vi "for_v0_v0.vi"() -> ()   [LabVIEW 2009]
panel:
  out "Numeric":dbl
  # "Afisare numere 0-24"
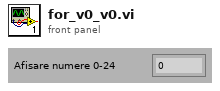
[diagram p1: front panel]
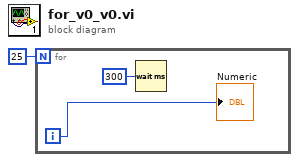
[diagram p0: block diagram]
diagram:
  n1 = for {
    N: 25 -> [_]
    i -> [w3]
    n2 = Wait (ms)(milliseconds to wait=u32 300) -> ()  [unwired: 1 out]
    "Numeric" <- w3
  }
